vi "Get Waveform Subset.vi"(11 "wfm in":waveform(dbl)) -> (3 "wfm out":waveform(dbl))   [LabVIEW 2021, in "Single Tone_DAC.lvlib"]
uses:
  Single Tone_DAC.lvlib
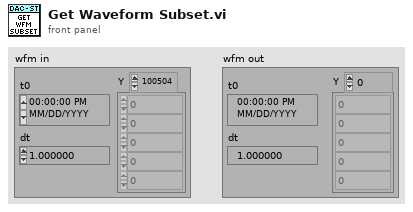
[diagram p1: front panel]
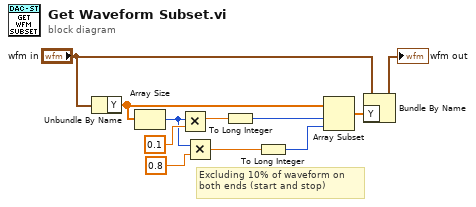
[diagram p0: block diagram]
diagram:
  # "Excluding 10% of waveform on\nboth ends (start and stop)"
  n1 = Unbundle By Name("wfm in") -> ("Y"=w8:dbl[])
  n2 = Array Size(array=w8) -> (size(s)=w5:i32)
  n3 = Multiply(x=w5, y=0.1) -> (x*y=w6:dbl)
  n4 = Multiply(x=w5, y=0.8) -> (x*y=w2:dbl)
  n5 = To Long Integer(number=w6) -> (32bit integer=w3:i32)
  n6 = To Long Integer(number=w2) -> (32bit integer=w1:i32)
  n7 = Array Subset(array=w8, index=w3, length=w1) -> (w9:dbl[])
  n8 = Bundle By Name(cluster="wfm in", "Y"=w9) -> (→"wfm out":waveform(dbl))
